vi "Get Types From Database.vi"(8 "error in (no error)":errorcluster, 10 "file?":bool, 11 "database":enum16{"dBase", "Jet", "SQL Server", "Oracle"}(ring)) -> (0 "error out":errorcluster, 3 "data types":string[](array[string]))   [LabVIEW 2011]
uses:
  <vilib>/addons/database/NI_Database_API.lvlib
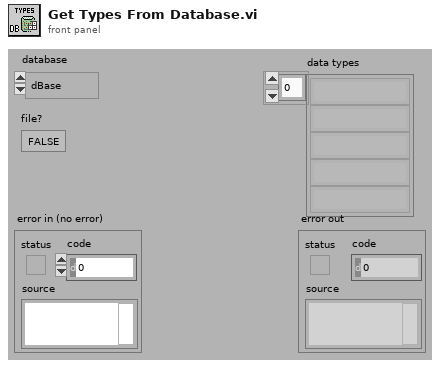
[diagram p1: front panel]
types:
  T1 = enum16{"varchar", "integer", "real", "float", "datetime", "image"}
  T2 = enum16{"varchar", "integer", "real", "float", "datetime", "oleobject"}
  T3 = enum16{"varchar", "integer", "real", "float", "date", "blob"}
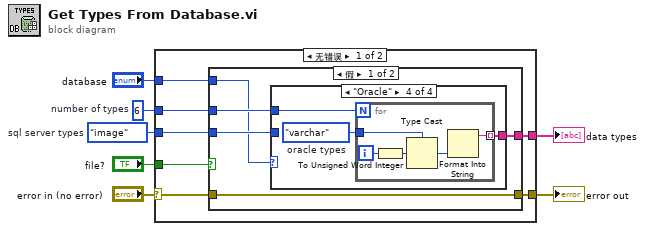
[diagram p0: block diagram]
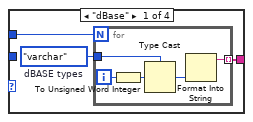
[diagram p2: hidden frame]
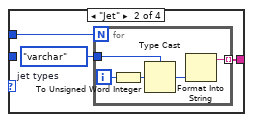
[diagram p3: hidden frame]
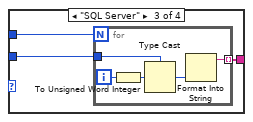
[diagram p4: hidden frame]
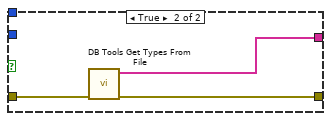
[diagram p5: hidden frame]
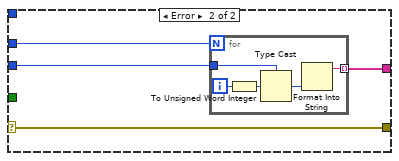
[diagram p6: hidden frame]
diagram:
  w4 = T1."image"  # sql server types
  w3 = 6  # number of types
  n1 = case shown="无错误" "error in (no error)" {
    selector: "error in (no error)" -> [w13 w58]
    tunnel: [w14 w58] -> w1
    tunnel: w3 -> [w12 w57]
    tunnel: w4 -> [w11 w56]
    tunnel: [w10 w55] -> w5
    tunnel: "database" -> [w9 _]
    tunnel: "file?" -> [w8 _]
    frame No Error {
      n2 = case shown="假" w8 {
        tunnel: w13 -> [w19 w54]
        tunnel: [w19 w53] -> w14
        tunnel: w12 -> [w18 _]
        tunnel: w11 -> [w16 _]
        tunnel: [w17 w52] -> w10
        tunnel: w9 -> [w15 _]
        frame False {
          n3 = case shown="\"Oracle\"" w15 {
            tunnel: w18 -> [w22 w30 w38 w46]
            tunnel: [w21 w29 w37 w45] -> w17
            tunnel: w16 -> [_ _ w36 _]
            frame "dBase" {
              w20 = T2."varchar"  # dBASE types
              n4 = for {
                N: w22 -> [_]
                tunnel: [w24] -> w21 mode=indexing
                tunnel: w20 -> [w23]
                i -> [w27]
                n5 = To Unsigned Word Integer(number=w27) -> (unsigned 16bit integer=w26:u16)
                n6 = Type Cast(type=w23, x=w26) -> (*(type *) &x=w25:T2)
                n7 = Format Into String(w25) -> (resulting string=w24:string)  [unwired: 3 in, 1 out]
              }
            }
            frame "Jet" {
              w28 = T2."varchar"  # jet types
              n8 = for {
                N: w30 -> [_]
                tunnel: [w32] -> w29 mode=indexing
                tunnel: w28 -> [w31]
                i -> [w35]
                n9 = To Unsigned Word Integer(number=w35) -> (unsigned 16bit integer=w34:u16)
                n10 = Type Cast(type=w31, x=w34) -> (*(type *) &x=w33:T2)
                n11 = Format Into String(w33) -> (resulting string=w32:string)  [unwired: 3 in, 1 out]
              }
            }
            frame "SQL Server" {
              n12 = for {
                N: w38 -> [_]
                tunnel: [w40] -> w37 mode=indexing
                tunnel: w36 -> [w39]
                i -> [w43]
                n13 = To Unsigned Word Integer(number=w43) -> (unsigned 16bit integer=w42:u16)
                n14 = Type Cast(type=w39, x=w42) -> (*(type *) &x=w41:T1)
                n15 = Format Into String(w41) -> (resulting string=w40:string)  [unwired: 3 in, 1 out]
              }
            }
            frame "Oracle" {
              w44 = T3."varchar"  # oracle types
              n16 = for {
                N: w46 -> [_]
                tunnel: [w48] -> w45 mode=indexing
                tunnel: w44 -> [w47]
                i -> [w51]
                n17 = To Unsigned Word Integer(number=w51) -> (unsigned 16bit integer=w50:u16)
                n18 = Type Cast(type=w47, x=w50) -> (*(type *) &x=w49:T3)
                n19 = Format Into String(w49) -> (resulting string=w48:string)  [unwired: 3 in, 1 out]
              }
            }
          }
        }
        frame True {
          n20 = call <vilib>:"DB Tools Get Types From File.vi"("error in (no error)"=w54) -> ("error out"=w53:errorcluster, "data types"=w52:string[])  [unwired: 5 in]
        }
      }
    }
    frame Error {
      n21 = for {
        N: w57 -> [_]
        tunnel: [w60] -> w55 mode=indexing
        tunnel: w56 -> [w59]
        i -> [w63]
        n22 = To Unsigned Word Integer(number=w63) -> (unsigned 16bit integer=w62:u16)
        n23 = Type Cast(type=w59, x=w62) -> (*(type *) &x=w61:T1)
        n24 = Format Into String(w61) -> (resulting string=w60:string)  [unwired: 3 in, 1 out]
      }
    }
  }
  "error out" <- w1
  "data types" <- w5
